vi "Read Local Dispatcher Port.vi"(11 "error in":errorcluster) -> (4 "UDP port":u16, 15 "error out":errorcluster)   [LabVIEW 2014, in "AMC.lvlib"]
doc: "Returns the UDP Port used by the local Dispatcher."
uses:
  AMC.lvlib
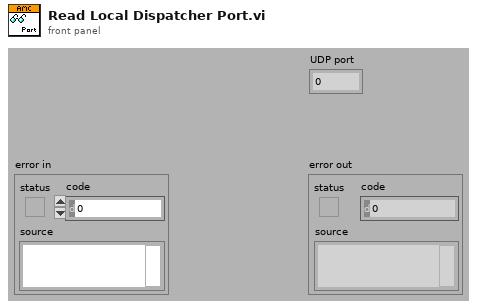
[diagram p1: front panel]
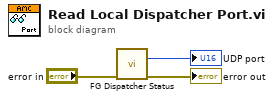
[diagram p0: block diagram]
diagram:
  n1 = call "FG Dispatcher Status.vi"("error in"="error in") -> ("UDP port out"=→"UDP port":u16, "error out"=→"error out":errorcluster)  [unwired: 12 in, 1 out]
